vi "ComplexCall.vi"(4 "Big":T2={"BigNumeric"=10.0, "BigBoolean"=TRUE, "BigString"="Insertale", "Small"={"SmallString"="Esto", "SmallNumeric"=20.0}}, 5 "Array":string[](array[string])=["Aqui", "Me", "Tienes", "Sufriendo", "Por", "Tu", "Culpa", "Llorando", "Sin", "Fin"], 6 "Numeric":dbl=-10.0, 7 "String":string="Voltealos") -> (0 "OutCluster":T1, 1 "Volteado":string[](array[string])=["Aqui", "Me", "Tienes", "Sufriendo", "Por", "Tu", "Culpa", "Llorando", "Sin", "Fin"], 2 "length":i32, 3 "concatenated string":string)   [LabVIEW 2010]
panel:
  in  "OutSmallCluster":cluster{"Numeric":dbl}
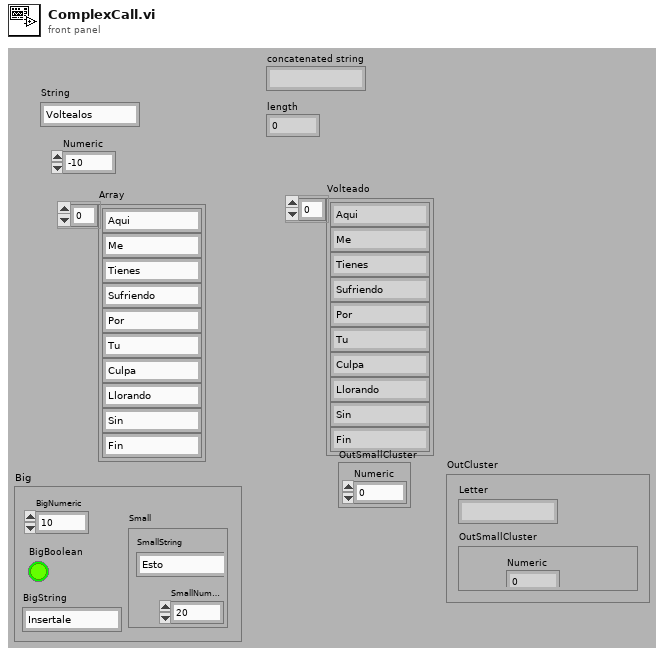
[diagram p1: front panel]
types:
  T1 = cluster{"Letter":string, "OutSmallCluster":cluster{"Numeric":dbl}}
  T2 = cluster{"BigNumeric":dbl, "BigBoolean":bool, "BigString":string, "Small":cluster{"SmallString":string, "SmallNumeric":dbl}}
  T3 = cluster{"SmallString":string, "SmallNumeric":dbl}
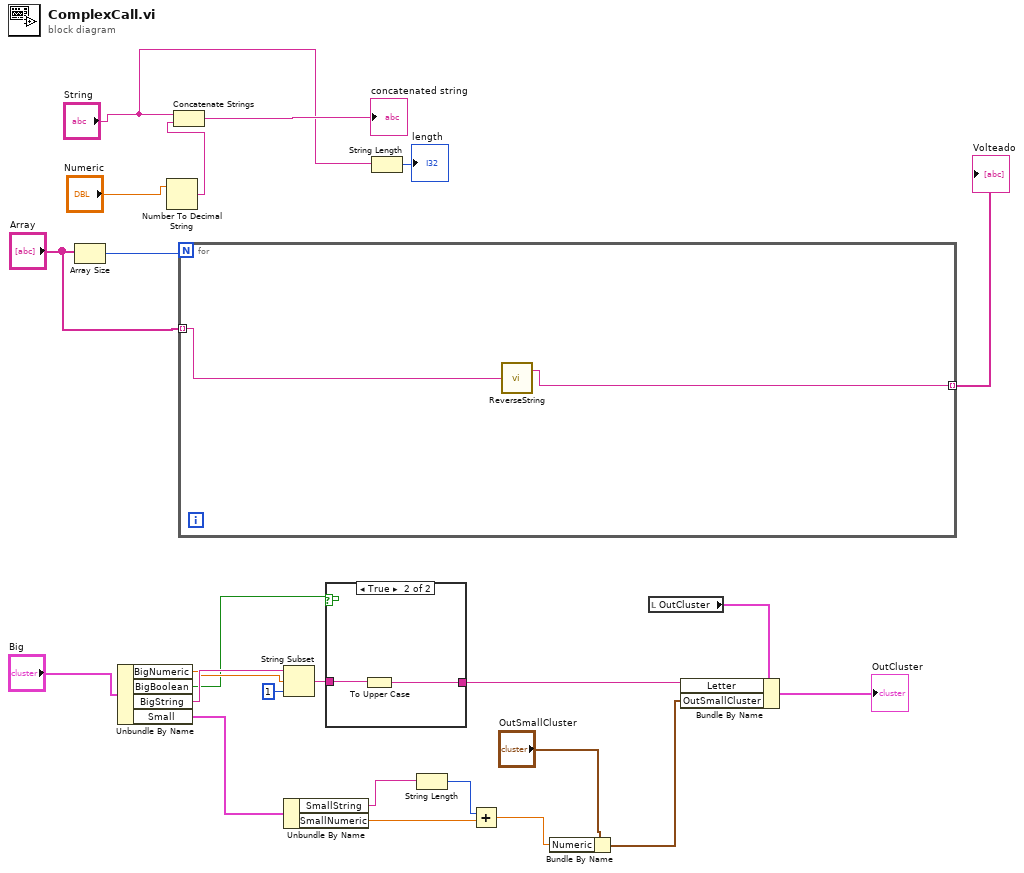
[diagram p0: block diagram]
diagram:
  n1 = Array Size(array="Array") -> (size(s)=w18:i32)
  n2 = Unbundle By Name("Big") -> ("BigNumeric"=w8:dbl, "BigBoolean"=w7:bool, "BigString"=w10:string, "Small"=w15:T3)
  n3 = Number To Decimal String(number="Numeric") -> (decimal integer string=w23:string)  [unwired: 1 out]
  n4 = Concatenate Strings("String", w23) -> (→"concatenated string":string)
  n5 = for {
    N: w18 -> [_]
    tunnel: "Array" -> [w26] mode=indexing
    tunnel: [w25] -> w17 mode=indexing
    n6 = call "ReverseString.vi"("InString"=w26) -> ("OutString"=w25:string)  [unwired: 1 out]
  }
  "Volteado" <- w17
  n7 = String Subset(string=w10, offset (0)=w8, length (rest)=1 ("length (rest)")) -> (substring=w6:string)
  n8 = Unbundle By Name(w15) -> ("SmallString"=w14:string, "SmallNumeric"=w12:dbl)
  n9 = case shown="True" w7 {
    tunnel: w6 -> [w27 w29]
    tunnel: [w27 w28] -> w5
    frame False {
    }
    frame True {
      n10 = To Upper Case(1:w29) -> (0:w28:string)
    }
  }
  n11 = String Length(string="String") -> (length=→"length":i32)
  n12 = String Length(string=w14) -> (length=w13:i32)
  n13 = Add(x=w13, y=w12) -> (x+y=w2:dbl)
  n14 = Bundle By Name(cluster="OutSmallCluster", "Numeric"=w2) -> (w1:cluster{"Numeric":dbl})
  n15 = local read "OutCluster"() -> (w11:T1)
  n16 = Bundle By Name(cluster=w11, "Letter"=w5, "OutSmallCluster"=w1) -> (→"OutCluster":T1)
